vi "PathPlanner_GeomUtil_CosineInterpolate.vi"(9 "T":dbl, 10 "EndVal":T1={"VALUE"=0.0, "COS"=1.0, "SIN"=0.0} {"SIN" format="%13.4f"; "COS" format="%13.4f"; "VALUE" format="%13.4f"}, 11 "StartVal":T1={"VALUE"=0.0, "COS"=1.0, "SIN"=0.0} {"SIN" format="%13.4f"; "COS" format="%13.4f"; "VALUE" format="%13.4f"}) -> (3 "InterpolatedValue":T1={"VALUE"=0.0, "COS"=1.0, "SIN"=0.0} {"SIN" format="%13.4f"; "COS" format="%13.4f"; "VALUE" format="%13.4f"})   [LabVIEW 2019, in "PathPlanner24.lvlib"]
doc: "Interpolate between two Rotation2ds\n \nInputs: \n - startVal - rotation2d - Start value\n - endVal - rotation2d - End value\n - t - double - Interpolation factor (0.0-1.0)\n\nOutputs:\n - Lerp - rotation2d - Interpolated value"
uses:
  <vilib>/Rock Robotics/WPI/ThirdParty/JAS_Junk/TrajLib/TypeDef/ROTATION2D.ctl
  <vilib>/Rock Robotics/WPI/ThirdParty/JAS_Junk/TrajLib/Rotation2d_UnaryMinus.vi
  <vilib>/Rock Robotics/WPI/ThirdParty/JAS_Junk/TrajLib/Rotation2d_RotateBy.vi
  <vilib>/Rock Robotics/WPI/ThirdParty/JAS_Junk/TrajLib/Rotation2d_CreateAngle.vi
  <vilib>/Rock Robotics/WPI/ThirdParty/JAS_Junk/TrajLib/Rotation2d_CreateXY.vi
  <vilib>/Rock Robotics/WPI/ThirdParty/JAS_Junk/TrajLib/Util_CalcDist.vi
  PathPlanner24.lvlib
  <vilib>/Rock Robotics/WPI/ThirdParty/JAS_Junk/TrajLib/Trajectory_Library.lvlib
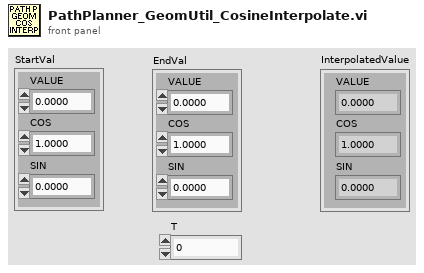
[diagram p1: front panel]
types:
  T1 = typedef "Trajectory_Library.lvlib/ROTATION2D.ctl" = cluster{"VALUE":dbl, "COS":dbl, "SIN":dbl}
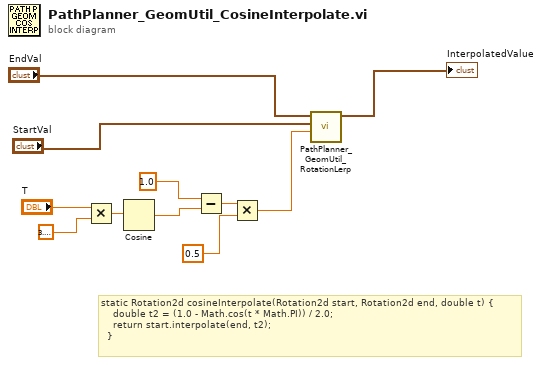
[diagram p0: block diagram]
diagram:
  # "static Rotation2d cosineInterpolate(Rotation2d start, Rotation2d end, double t) {\n    double t2 = (1.0 - Math.cos(t * Math.PI)) / 2.0;\n    return start.interpolate(end, t2);\n  }"
  n1 = Multiply(x="T", y=3.141592653589793) -> (x*y=w9:dbl)
  n2 = Cosine(x=w9) -> (cos(x)=w7:dbl)
  n3 = Subtract(x=1.0, y=w7) -> (x-y=w6:dbl)
  n4 = Multiply(x=w6, y=0.5) -> (x*y=w2:dbl)
  n5 = call "PathPlanner_GeomUtil_RotationLerp.vi"("T"=w2, "EndVal"="StartVal", "StartVal"="EndVal") -> ("Lerp"=→"InterpolatedValue":T1)  [unwired: 8 in]
